vi "is UTF-8.vi"(11 "String":string) -> (3 "UTF8":bool)   [LabVIEW 2017]
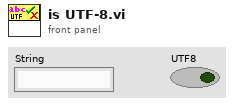
[diagram p1: front panel]
types:
  T1 = enum16{"Safe", "Non-En First Char Found", "Match UTF-8"}
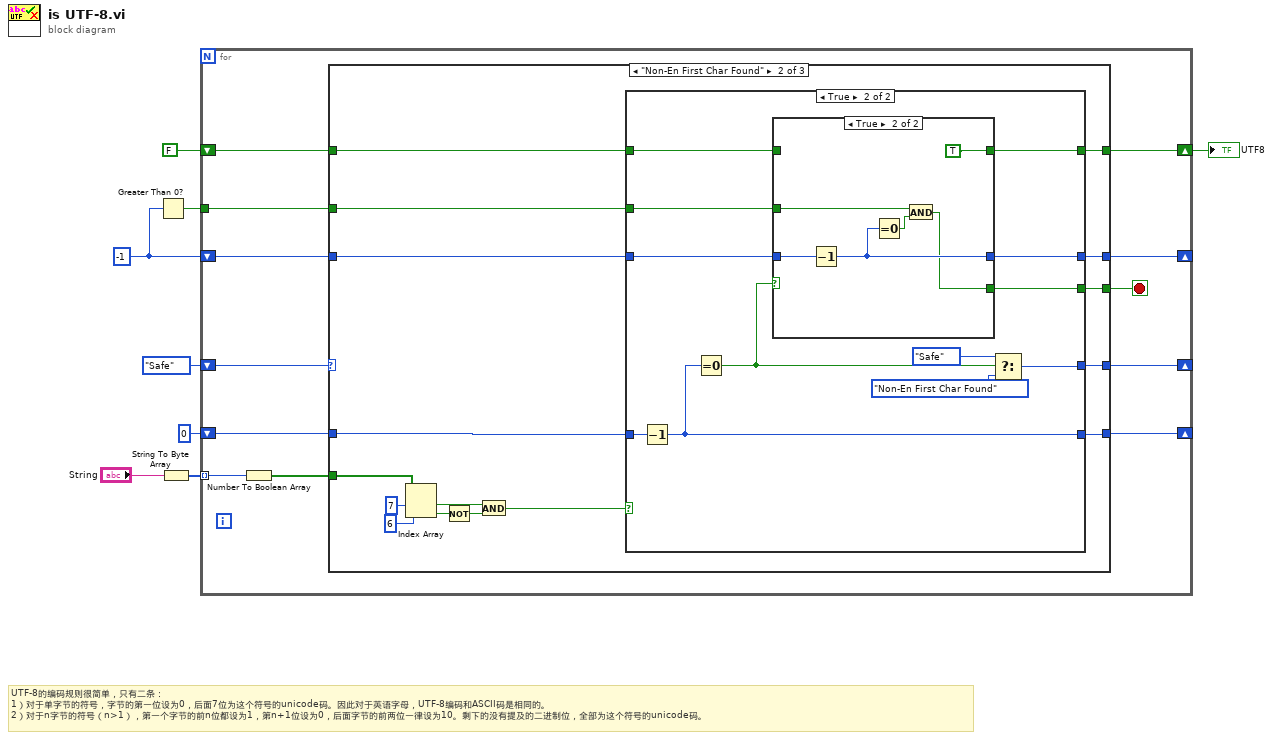
[diagram p0: block diagram]
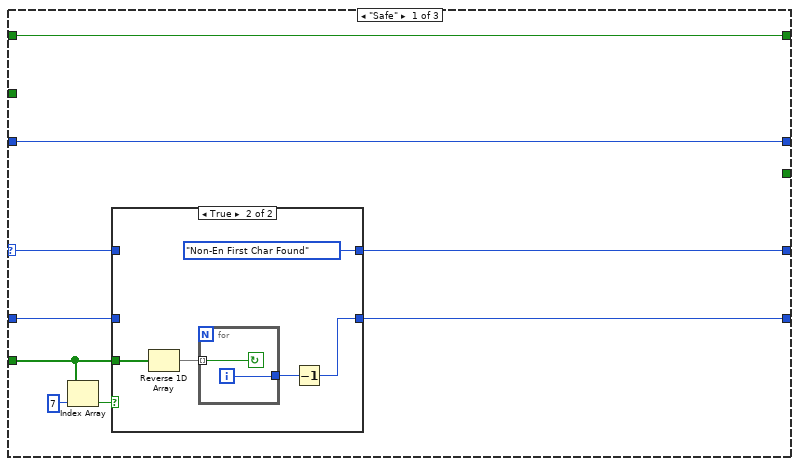
[diagram p2: hidden frame]
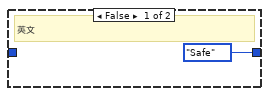
[diagram p3: hidden frame]
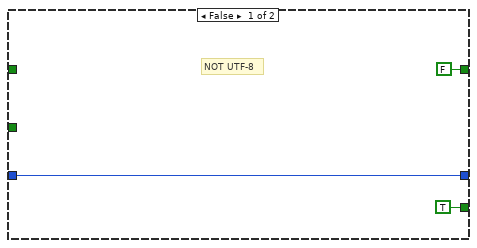
[diagram p4: hidden frame]
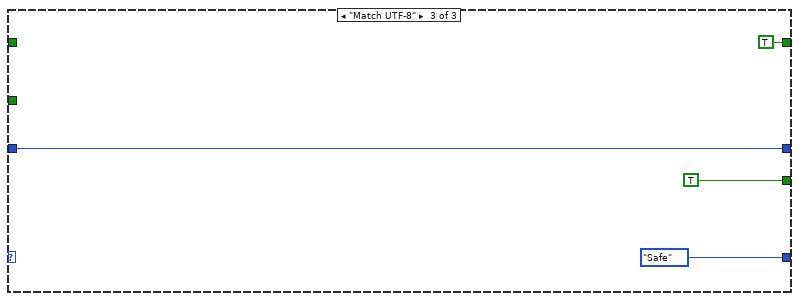
[diagram p6: hidden frame]
diagram:
  w5 = -1
  # "UTF-8的编码规则很简单，只有二条：\n1）对于单字节的符号，字节的第一位设为0，后面7位为这个符号的unicode码。因此对于英语字母，UTF-8编码和ASCII码是相同的。\n2）对于n字节的符号（n>1），第一个字节的前n位都设为1，第n+1位设为0，后面字节的前两位一律设为10。剩下的没有提及的二进制位，全部为这个符号的unicode码。"
  n1 = Greater Than 0?(x=w5) -> (x > 0?=w6:bool)
  n2 = String To Byte Array(string="String") -> (unsigned byte array=w2:u8[])
  n3 = for {
    shift-right: [w18] -> _
    shift-left: T1."Safe" -> [w19]
    shift-right: [w17] -> _
    shift-left: 0 -> [w16]
    tunnel: w2 -> [w11] mode=indexing
    shift-right: [w15] -> _
    shift-left: w5 -> [w14]
    tunnel: w6 -> [w12]
    shift-right: [w9] -> w8
    shift-left: FALSE ("UTF8") -> [w10]
    stop <- w13 stop-if-true
    n4 = Number To Boolean Array(number=w11) -> (Boolean array=w20:bool[])
    n5 = case shown="\"Non-En First Char Found\"" w19 {
      selector: w19 -> [w27 _ _]
      tunnel: w20 -> [w25 w52 _]
      tunnel: [w26 w48 T1."Safe" ("f")] -> w18
      tunnel: [w24 w47 _] -> w17
      tunnel: w16 -> [w23 w49 _]
      tunnel: [_ w44 TRUE] -> w13
      tunnel: [w22 w46 w78] -> w15
      tunnel: w14 -> [w22 w45 w78]
      tunnel: w12 -> [_ w43 _]
      tunnel: w10 -> [w21 w39 _]
      tunnel: [w21 w38 TRUE ("UTF8")] -> w9
      frame "Safe" {
        n6 = Index Array(array=w25, index=7) -> (element=w28:bool)
        n7 = case shown="True" w28 {
          tunnel: w27 -> [_ _]
          tunnel: [T1."Safe" T1."Non-En First Char Found"] -> w26
          tunnel: w25 -> [_ w34]
          tunnel: [_ w31] -> w24
          tunnel: w23 -> [_ _]
          frame False {
            # "英文"
          }
          frame True {
            n8 = Reverse 1D Array(array=w34) -> (reversed array=w33:bool[])
            n9 = for {
              tunnel: w33 -> [w37] mode=indexing
              tunnel: [w36] -> w32
              i -> [w36]
              stop <- w37 continue-if-true
            }
            n10 = Decrement(x=w32) -> (x-1=w31:i32)
          }
        }
      }
      frame "Non-En First Char Found" {
        n11 = Index Array(array=w52, index #1=7 ("index"), index #2=6 ("index")) -> (element #1=w42:bool, element #2=w50:bool)
        n12 = Not(x=w50) -> (.not. x?=w40:bool)
        n13 = And(x=w42, y=w40) -> (x .and. y?=w41:bool)
        n14 = case shown="True" w41 {
          tunnel: w49 -> [_ w68]
          tunnel: [_ w66] -> w48
          tunnel: [_ w62] -> w47
          tunnel: [w56 w64] -> w46
          tunnel: w45 -> [w56 w63]
          tunnel: [TRUE w59] -> w44
          tunnel: w43 -> [_ w60]
          tunnel: w39 -> [_ w58]
          tunnel: [FALSE ("UTF8") w57] -> w38
          frame False {
            # "NOT UTF-8"
          }
          frame True {
            n15 = Decrement(x=w68) -> (x-1=w62:i32)
            n16 = Equal To 0?(x=w62) -> (x = 0?=w65:bool)
            n17 = case shown="True" w65 {
              tunnel: [w70 w74] -> w64
              tunnel: w63 -> [w70 w76]
              tunnel: w60 -> [_ w73]
              tunnel: [_ w72] -> w59
              tunnel: w58 -> [w69 _]
              tunnel: [w69 TRUE ("UTF8")] -> w57
              frame False {
              }
              frame True {
                n18 = Decrement(x=w76) -> (x-1=w74:i32)
                n19 = Equal To 0?(x=w74) -> (x = 0?=w75:bool)
                n20 = And(x=w73, y=w75) -> (x .and. y?=w72:bool)
              }
            }
            n21 = Select(t=T1."Safe", s=w65, f=T1."Non-En First Char Found") -> (s? t:f=w66:T1)
          }
        }
      }
      frame "Match UTF-8" {
      }
    }
  }
  "UTF8" <- w8
